vi "deleteObserver.vi"(8 "error in (no error)":errorcluster, 10 "index":u16, 11 "Observable in":refnum<class "Observable.lvclass">) -> (0 "error out":errorcluster, 3 "Observable out":refnum<class "Observable.lvclass">)   [LabVIEW 2020, in "Observable.lvclass"]
uses:
  Observable.lvclass
  Observable.lvclass/Observable.ctl
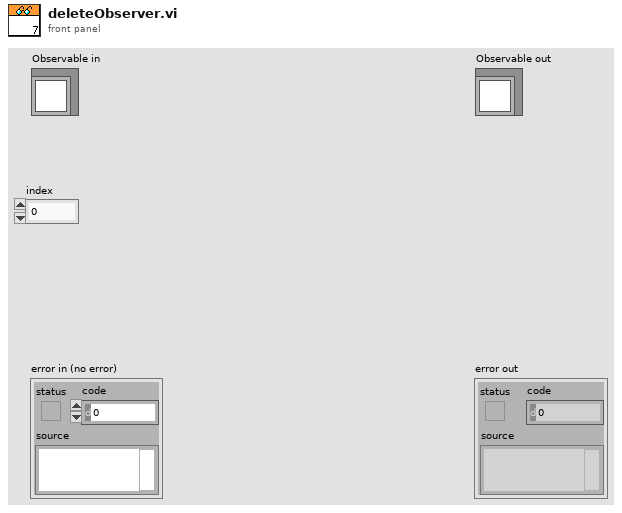
[diagram p1: front panel]
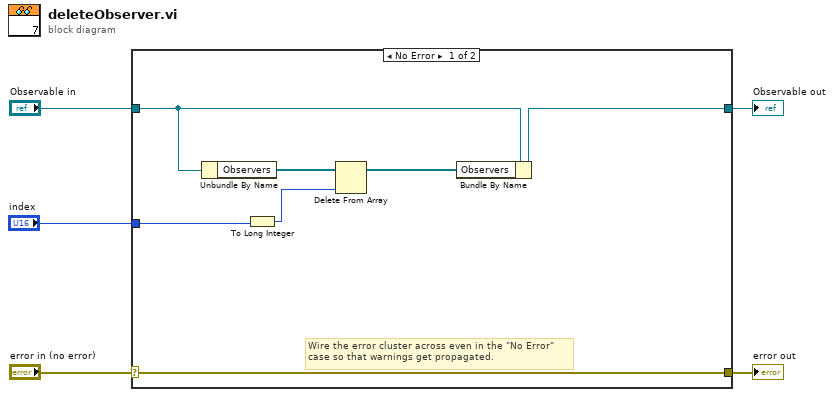
[diagram p0: block diagram]
diagram:
  n1 = case shown="No Error" "error in (no error)" {
    selector: "error in (no error)" -> [w12 w14]
    tunnel: [w12 w14] -> w4
    tunnel: [w9 w13] -> w2
    tunnel: "Observable in" -> [w11 w13]
    tunnel: "index" -> [w7 _]
    frame No Error {
      # "Wire the error cluster across even in the \"No Error\"\ncase so that warnings get propagated."
      n2 = Unbundle By Name(w11) -> ("Observers"=w10:refnum<class "Observer.lvclass">[])
      n3 = To Long Integer(number=w7) -> (32bit integer=w6:i32)
      n4 = Delete From Array(array=w10, index=w6) -> (array with subset deleted=w8:refnum<class "Observer.lvclass">[])  [unwired: 1 in, 1 out]
      n5 = Bundle By Name(cluster=w11, "Observers"=w8) -> (w9:refnum<class "Observable.lvclass">)
    }
    frame Error {
    }
  }
  "error out" <- w4
  "Observable out" <- w2
